vi "ClusterDataTypeToTagBusDataType.vi"(10 "Array Type":T1, 11 "Type Enum":T1) -> (3 "data type":T2)   [LabVIEW 2013, in "control module data interface generator.lvlib"]
uses:
  control module data interface generator.lvlib
  <vilib>/Utility/VariantDataType/Type.ctl
  <vilib>/NI/Tag Bus/tag/Data Type.ctl
  <vilib>/NI/Tag Bus/tag/tag descriptor.lvclass
  <vilib>/Utility/VariantDataType/VariantType.lvlib
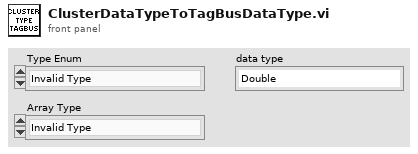
[diagram p1: front panel]
types:
  T1 = typedef "VariantType.lvlib/Type.ctl" = enum8{"Invalid Type", "Void", "I8", "I16", "I32", "I64", "U8", "U16", "U32", "U64", "Single Float", "Double Float", "Extended Float", "Single Complex", "Double Complex", "Extended Complex", "Enum U8", "Enum U16", "Enum U32", "Enum U64", "Single Float With Unit", "Double Float With Unit", "Extended Float With Unit", "Single Complex with Unit", "Double Complex with Unit", "Extended Complex with Unit", "Boolean", "String", "Path", "Picture", "Tag", "Array", "Cluster", "Variant", "LV Variant", "Waveform", "Timestamp", "Digital Waveform", "Digital Data", "ExpressData", "Refnum", "External Data", "VI", "Poly VI", "LabVIEW Class Instance", "Fixed Point"}
  T2 = typedef "tag bus.lvlib/tag descriptor.lvclass/Data Type.ctl" = enum16{"Double", "Single", "I64", "I32", "I16", "I8", "U64", "U32", "U16", "U8", "Boolean", "String", "Array of Double", "Array of Single", "Array of I64", "Array of I32", "Array of I16", "Array of I8", "Array of U64", "Array of U32", "Array of U16", "Array of U8", "Array of Boolean", "Array of String"}
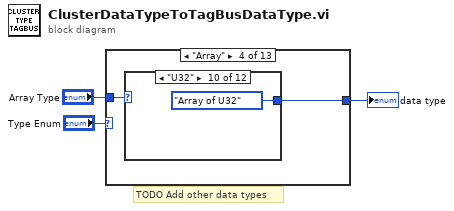
[diagram p0: block diagram]
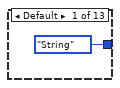
[diagram p2: hidden frame]
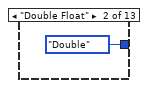
[diagram p3: hidden frame]
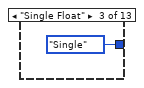
[diagram p4: hidden frame]
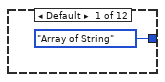
[diagram p5: hidden frame]
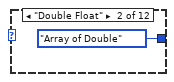
[diagram p6: hidden frame]
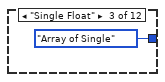
[diagram p7: hidden frame]
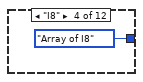
[diagram p8: hidden frame]
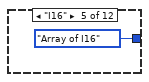
[diagram p9: hidden frame]
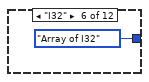
[diagram p10: hidden frame]
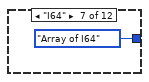
[diagram p11: hidden frame]
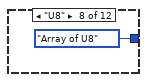
[diagram p12: hidden frame]
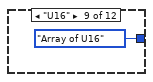
[diagram p13: hidden frame]
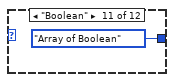
[diagram p14: hidden frame]
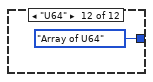
[diagram p15: hidden frame]
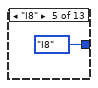
[diagram p16: hidden frame]
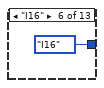
[diagram p17: hidden frame]
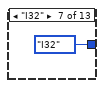
[diagram p18: hidden frame]
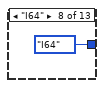
[diagram p19: hidden frame]
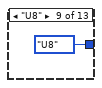
[diagram p20: hidden frame]
diagram:
  # "TODO Add other data types"
  n1 = case shown="\"Array\"" "Type Enum" {
    tunnel: [Data_Type."String" ("data type") Data_Type."Double" ("data type") Data_Type."Single" ("data type") w7 Data_Type."I8" ("data type") Data_Type."I16" ("data type") Data_Type."I32" ("data type") Data_Type."I64" ("data type") Data_Type."U8" ("data type") Data_Type."U16" ("data type") Data_Type."U32" ("data type") Data_Type."Boolean" ("data type") Data_Type."U64" ("data type")] -> w2
    tunnel: "Array Type" -> [_ _ _ w8 _ _ _ _ _ _ _ _ _]
    frame Default {
    }
    frame "Double Float" {
    }
    frame "Single Float" {
    }
    frame "Array" {
      n2 = case shown="\"U32\"" w8 {
        tunnel: [Data_Type."Array of String" ("data type") Data_Type."Array of Double" ("data type") Data_Type."Array of Single" ("data type") Data_Type."Array of I8" ("data type") Data_Type."Array of I16" ("data type") Data_Type."Array of I32" ("data type") Data_Type."Array of I64" ("data type") Data_Type."Array of U8" ("data type") Data_Type."Array of U16" ("data type") Data_Type."Array of U32" ("data type") Data_Type."Array of Boolean" ("data type") Data_Type."Array of U64" ("data type")] -> w7
        frame Default {
        }
        frame "Double Float" {
        }
        frame "Single Float" {
        }
        frame "I8" {
        }
        frame "I16" {
        }
        frame "I32" {
        }
        frame "I64" {
        }
        frame "U8" {
        }
        frame "U16" {
        }
        frame "U32" {
        }
        frame "Boolean" {
        }
        frame "U64" {
        }
      }
    }
    frame "I8" {
    }
    frame "I16" {
    }
    frame "I32" {
    }
    frame "I64" {
    }
    frame "U8" {
    }
    frame "U16" {
    }
    frame "U32" {
    }
    frame "Boolean" {
    }
    frame "U64" {
    }
  }
  "data type" <- w2
